vi "SFOAE-Initialize.vi"(0 "SFOAE":T4, 1 "State":T1, 5 "OAEPhsRef":refnum<vi>, 7 "OAEMagRef":refnum<vi>, 9 "StimMagRef":refnum<vi>) -> (3 "Expt State out":T1, 4 "AO Runtime":T3, 8 "DataProc":T2, 15 "error out":errorcluster)   [LabVIEW 2020]
uses:
  Typedefs/SFOAE-Parameters.ctl
  Typedefs/SFOAE-Stimulus Parameters.ctl
  Typedefs/SFOAE-Sweep Params.ctl
  Typedefs/SFOAE-Response Parameters.ctl
  Typedefs/SFOAE-AO Runtime Data.ctl
  CFTS Main Panel SubVIs/CFTS-Experiment State.ctl
  Typedefs/SFOAE-Data Processing.ctl
  epl-vi-lib/Connection VIs/Type Defs/Input sources.ctl
  epl-vi-lib/Connection VIs/Type Defs/Output sources.ctl
panel:
  in  "Frame size (s)":dbl=0.5
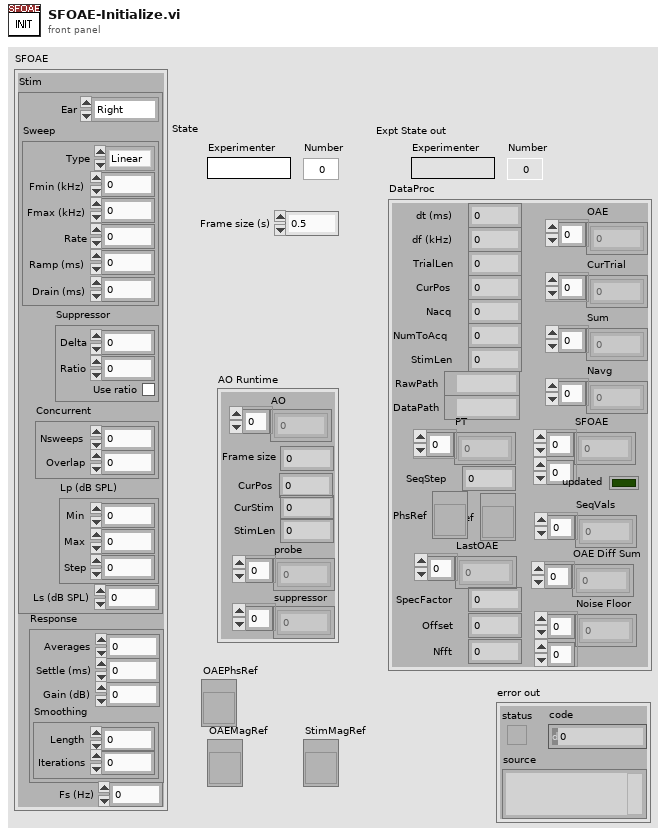
[diagram p1: front panel]
types:
  T1 = typedef "CFTS-Experiment State.ctl" = cluster{"Experimenter":string, "Number":u32, "Right":string, "Left":string, "Data Folder":path, "State File":path, "Version Info":string, "End Exposure Time":dbl, "Exposure Duration":string, "Run #":cluster{"CAP":i16, "ABR":i16, "DP":i16, "VsEP":i16, "MeasSeq":i16, "SubSeq":i16, "SFOAE":i16}}
  T2 = typedef "SFOAE-Data Processing.ctl" = cluster{"dt (ms)":dbl, "TrialLen":i32, "PT":cdb[], "CurPos":i32, "Sum":dbl[], "Navg":dbl[], "Nacq":i32, "RawPath":path, "DataPath":path, "NumToAcq":i32, "OAE":dbl[], "CurTrial":dbl[], "StimLen":i32, "SFOAE":cdb[][], "SeqStep":i32, "updated":bool, "SeqVals":dbl[], "df (kHz)":dbl, "MagRef":refnum<vi>, "LastOAE":dbl[], "OAE Diff Sum":dbl[], "Noise Floor":cdb[][], "SpecFactor":dbl, "Offset":i32, "Nfft":i32, "PhsRef":refnum<vi>}
  T3 = typedef "SFOAE-AO Runtime Data.ctl" = cluster{"AO":i32[], "Frame size":i32, "CurPos":i32, "probe":dbl[], "suppressor":dbl[], "CurStim":i32, "StimLen":i32}
  T4 = typedef "SFOAE-Parameters.ctl" = cluster{"Stim":T5, "Response":T7, "Fs (Hz)":dbl}
  T5 = typedef "SFOAE-Stimulus Parameters.ctl" = cluster{"Ear":enum16{"Right", "Left"}, "Sweep":T6, "Suppressor":cluster{"Delta":dbl, "Ratio":dbl, "Use ratio":bool}, "Concurrent":cluster{"Nsweeps":i32, "Overlap":dbl}, "Ls (dB SPL)":dbl, "Lp (dB SPL)":cluster{"Min":dbl, "Max":dbl, "Step":dbl}}
  T6 = typedef "SFOAE-Sweep Params.ctl" = cluster{"Type":enum16{"Linear", "Log"}, "Fmin (kHz)":dbl, "Fmax (kHz)":dbl, "Rate":dbl, "Ramp (ms)":dbl, "Drain (ms)":dbl}
  T7 = typedef "SFOAE-Response Parameters.ctl" = cluster{"Averages":i32, "Settle (ms)":dbl, "Gain (dB)":dbl, "Smoothing":cluster{"Length":i32, "Iterations":i32}}
  T8 = typedef "Output sources.ctl" = u16
  T9 = typedef "Input sources.ctl" = u16
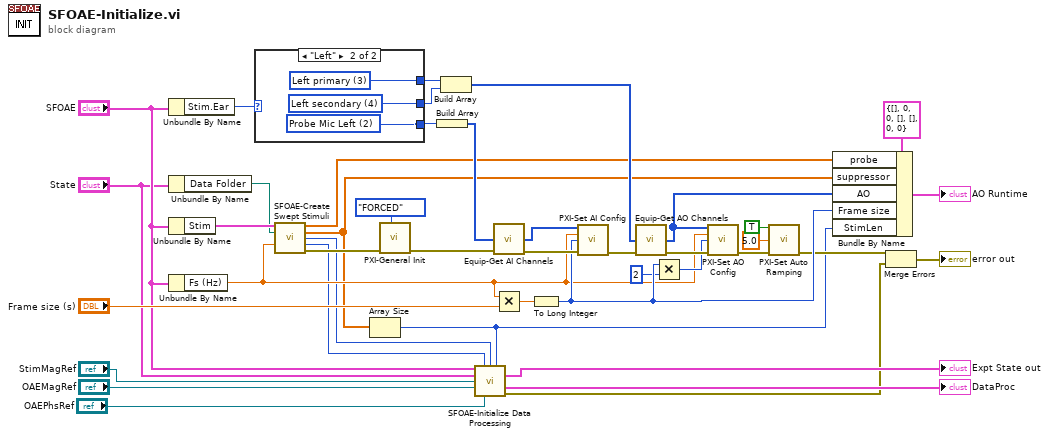
[diagram p0: block diagram]
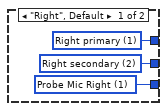
[diagram p2: hidden frame]
diagram:
  n1 = Unbundle By Name("SFOAE") -> ("Stim.Ear"=w42:enum16{"Right", "Left"})
  n2 = Unbundle By Name("State") -> ("Data Folder"=w23:path)
  n3 = Unbundle By Name("SFOAE") -> ("Stim"=w28:T5)
  n4 = Unbundle By Name("SFOAE") -> ("Fs (Hz)"=w17:dbl)
  n5 = case shown="\"Left\"" w42 {
    tunnel: [w45 w48] -> w41
    tunnel: [w44 w47] -> w35
    tunnel: [w43 w46] -> w34
    frame "Right", Default {
      w43 = T8 2 items=["--unused--", "Right primary", "Right secondary", "Left primary", "Left secondary", "Shocks", "Startle", "Background", "Shaker", "Blue laser"] ("Ring")
      w44 = T8 1 items=["--unused--", "Right primary", "Right secondary", "Left primary", "Left secondary", "Shocks", "Startle", "Background", "Shaker", "Blue laser"] ("Ring")
      w45 = T9 1 items=["--unused--", "Probe Mic Right", "Probe Mic Left", "Cal Mic", "ABR", "CAP Right", "CAP Left", "Startle piezo", "Temperature", "Heart rate", "Accelerometer", "Startle piezo 2"] ("Ring")
    }
    frame "Left" {
      w46 = T8 4 items=["--unused--", "Right primary", "Right secondary", "Left primary", "Left secondary", "Shocks", "Startle", "Background", "Shaker", "Blue laser"] ("Ring")
      w47 = T8 3 items=["--unused--", "Right primary", "Right secondary", "Left primary", "Left secondary", "Shocks", "Startle", "Background", "Shaker", "Blue laser"] ("Ring")
      w48 = T9 2 items=["--unused--", "Probe Mic Right", "Probe Mic Left", "Cal Mic", "ABR", "CAP Right", "CAP Left", "Startle piezo", "Temperature", "Heart rate", "Accelerometer", "Startle piezo 2"] ("Ring")
    }
  }
  n6 = call "SFOAE-Create Swept Stimuli.vi"("SFOAE Stim"=w28, "Data Folder"=w23, "Fs (Hz)"=w17) -> ("probe"=w21:dbl[], "suppressor"=w16:dbl[], "offset"=w3:i32, "nfft"=w2:i32, "error out"=w27:errorcluster)  [unwired: 8 in]
  n7 = Array Size(array=w16) -> (size(s)=w4:i32)
  n8 = call "PXI-General Init.vi"("Double Buffer Mode"=enum32{"OFF", "ENABLED", "FORCED"}."FORCED", "error in (no error)"=w27) -> ("error out"=w40:errorcluster)  [unwired: 9 in]
  n9 = Build Array(w41) -> (w39:T9[])
  n10 = Build Array(w35, w34) -> (w33:T8[])
  n11 = call "SFOAE-Initialize Data Processing.vi"("SFOAE"="SFOAE", "nfft"=w2, "offset"=w3, "StimLen"=w4, "State"="State", "StimMagRef"="StimMagRef", "OAEMagRef"="OAEMagRef", "OAEPhsRef"="OAEPhsRef") -> ("Expt State out"=→"Expt State out":T1, "DataProc"=→"DataProc":T2, "error out"=w8:errorcluster)  [unwired: 5 in]
  n12 = call "Equip-Get AI Channels.vi"("Inputs"=w39, "error in (no error)"=w40) -> ("AI Channels"=w38:i32[], "error out"=w37:errorcluster)  [unwired: 12 in]
  n13 = Multiply(x=w17, y="Frame size (s)") -> (x*y=w29:dbl)
  n14 = To Long Integer(number=w29) -> (32bit integer=w20:i32)
  n15 = call "PXI-Set AI Config.vi"("AI Channels"=w38, "Sampling Rate (Hz)"=w17, "Buffer Size"=w20, "error in (no error)"=w37) -> ("error out"=w36:errorcluster)  [unwired: 11 in]
  n16 = call "Equip-Get AO Channels.vi"("Outputs"=w33, "error in (no error)"=w36) -> ("AO Channels"=w26:i32[], "error out"=w32:errorcluster)  [unwired: 12 in]
  n17 = Multiply(x=w20, y=2) -> (x*y=w18:i32)
  n18 = call "PXI-Set AO Config.vi"("AO Channels"=w26, "Sampling Rate (Hz)"=w17, "Buffer Size"=w18, "error in (no error)"=w32) -> ("error out"=w22:errorcluster)  [unwired: 11 in]
  n19 = call "PXI-Set Auto Ramping.vi"("Auto ramp?"=TRUE, "Ramp duration (ms)"=5.0, "error in (no error)"=w22) -> ("error out"=w10:errorcluster)  [unwired: 12 in]
  n20 = Bundle By Name(cluster=T3 {"AO"=[], "Frame size"=0, "CurPos"=0, "probe"=[], "suppressor"=[], "CurStim"=0, "StimLen"=0} ("AO Runtime"), "probe"=w21, "suppressor"=w16, "AO"=w26, "Frame size"=w20, "StimLen"=w4) -> (→"AO Runtime":T3)
  n21 = Merge Errors(w10, w8) -> (→"error out":errorcluster)
